vi "AK8963-measurement Data process.vi"(7 "ASA":u8[](array[numeric]), 8 "error in":errorcluster, 11 "Bytes Read":u8[](array[numeric])) -> (0 "error OUT":errorcluster, 2 "measure":dbl[](array[numeric]))   [LabVIEW 2019]
uses:
  <vilib>/Utility/error.llb/Error Cluster From Error Code.vi
  <vilib>/ErrorRing/Error Ring.xnode
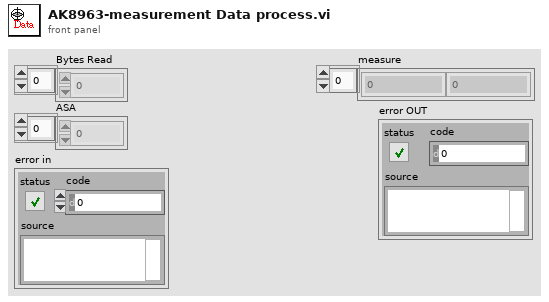
[diagram p1: front panel]
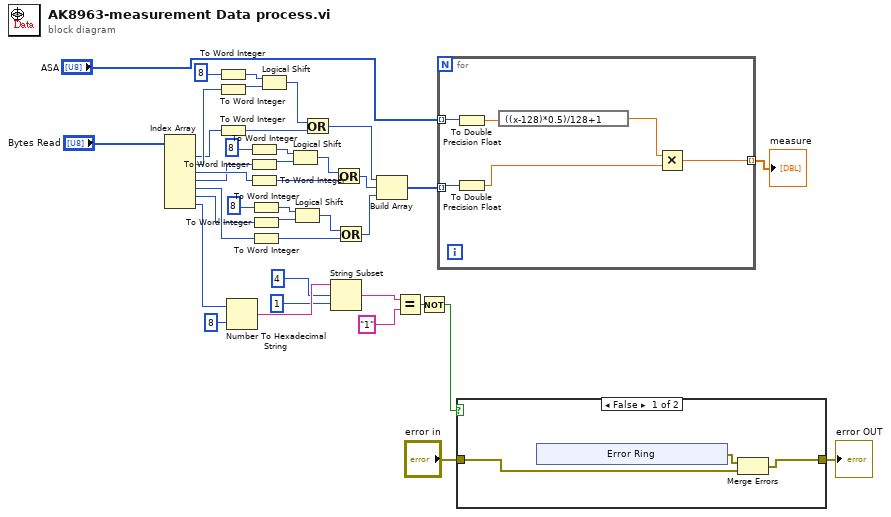
[diagram p0: block diagram]
diagram:
  n1 = Index Array(array="Bytes Read") -> (element #1=w35:u8, element #2=w36:u8, element #3=w22:u8, element #4=w21:u8, element #5=w20:u8, element #6=w19:u8, element #7=w15:u8)  [unwired: 7 in]
  n2 = To Word Integer(number=8) -> (16bit integer=w38:i16)
  n3 = To Word Integer(number=w36) -> (16bit integer=w37:i16)
  n4 = To Word Integer(number=w35) -> (16bit integer=w33:i16)
  n5 = Number To Hexadecimal String(1:i16 8 ("width (-)"), 2:w15) -> (0:w17:string)
  n6 = To Word Integer(number=8) -> (16bit integer=w29:i16)
  n7 = To Word Integer(number=w21) -> (16bit integer=w30:i16)
  n8 = To Word Integer(number=w22) -> (16bit integer=w32:i16)
  n9 = To Word Integer(number=8) -> (16bit integer=w26:i16)
  n10 = To Word Integer(number=w19) -> (16bit integer=w25:i16)
  n11 = To Word Integer(number=w20) -> (16bit integer=w23:i16)
  n12 = Logical Shift(y=w38, x=w37) -> (x << y=w34:i16)
  n13 = Logical Shift(y=w29, x=w30) -> (x << y=w31:i16)
  n14 = Logical Shift(y=w26, x=w25) -> (x << y=w24:i16)
  n15 = Or(x=w34, y=w33) -> (x .or. y?=w9:i16)
  n16 = String Subset(string=w17, offset (0)=4, length (rest)=1 ("offset (0)")) -> (substring=w13:string)
  n17 = Or(x=w31, y=w32) -> (x .or. y?=w10:i16)
  n18 = Or(x=w24, y=w23) -> (x .or. y?=w8:i16)
  n19 = Build Array(w9, w10, w8) -> (w7:i16[])
  n20 = Equal?(x=w13, y="1") -> (x = y?=w4:bool)
  n21 = Not(x=w4) -> (.not. x?=w1:bool)
  n22 = for {
    tunnel: w7 -> [w44] mode=indexing
    tunnel: "ASA" -> [w45] mode=indexing
    tunnel: [w40] -> w5 mode=indexing
    n23 = To Double Precision Float(number=w45) -> (double precision float=w43:dbl)
    n24 = To Double Precision Float(number=w44) -> (double precision float=w42:dbl)
    n25 = expression code="((x-128)*0.5)/128+1"(w43) -> (w41:dbl)
    n26 = Multiply(x=w41, y=w42) -> (x*y=w40:dbl)
  }
  "measure" <- w5
  n27 = case shown="False" w1 {
    tunnel: [w48 w54] -> w2
    tunnel: "error in" -> [w46 w54]
    frame False {
      n28 = xnode "Error Ring"() -> ("error out"=w47:errorcluster)
      n29 = Merge Errors(w47, w46) -> (w48:errorcluster)
    }
    frame True {
    }
  }
  "error OUT" <- w2
